vi "add-subhiearchy.vi"(6 "appended path":path, 8 "all relative paths":path[](array[path]), 9 "indices of kept elements":i32[](array[numeric]), 10 "tree main structure":string[](array[string]), 11 "all vi paths":path[](array[path])) -> ()   [LabVIEW 2014]
uses:
  controls/state-machine.ctl
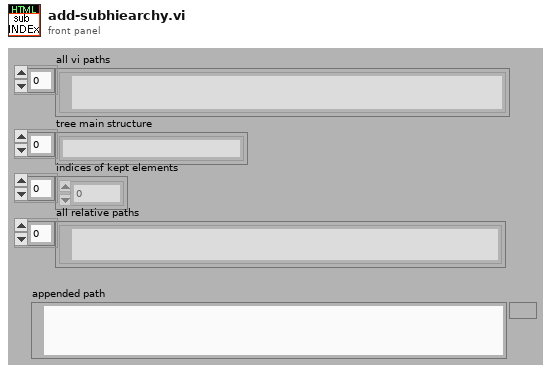
[diagram p1: front panel]
types:
  T1 = typedef "state-machine.ctl" = enum16{"add carridge return", "init", "Read-inputs", "edit generated file", "end", "Add front panel", "Add Block Diagram", "Add VI icon", "Add VI description", "Add VI hiearchy", "Add list of sub vis", "add custom html", "open report in browser", "Save report to file", "dispose report", "Add header text", "Create style .css", "add-red-box-header", "Delete Temp Files", "Remove-path-element", "add-revision-history", "add-icon-image-only"}
  T2 = typedef "state program.ctl" = cluster{"State machine":T1, "HTML before":string, "HTML after":string}
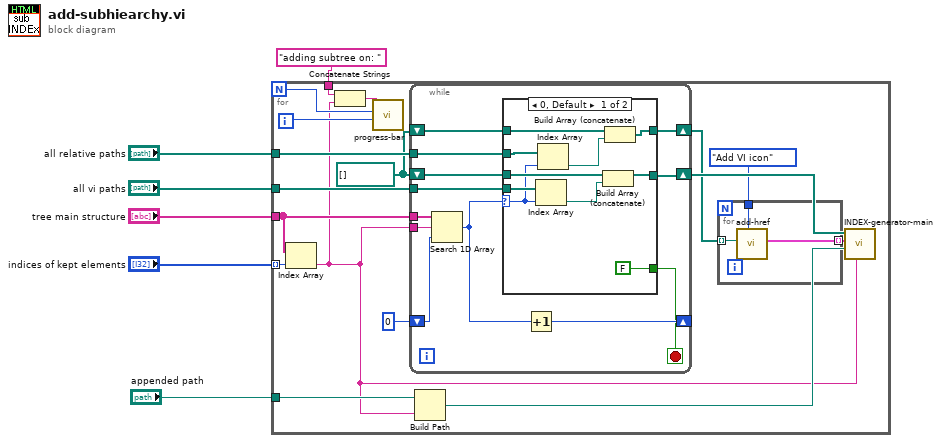
[diagram p0: block diagram]
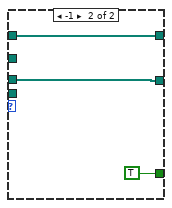
[diagram p2: hidden frame]
diagram:
  n1 = for {
    N -> [w12]
    tunnel: "tree main structure" -> [w22]
    tunnel: "indices of kept elements" -> [w23] mode=indexing
    tunnel: "all vi paths" -> [w21]
    tunnel: "all relative paths" -> [w19]
    tunnel: "appended path" -> [w15]
    tunnel: "adding subtree on: " -> [w8]
    i -> [w11]
    w18 = path[] []
    n2 = Index Array(array=w22, index=w23) -> (element=w9:string)
    n3 = Concatenate Strings(w8, w9) -> (w10:string)
    n4 = call "progress-bar.vi"("i++"=w11, "max"=w12, "state"=w10) -> ()  [unwired: 9 out]
    n5 = while {
      tunnel: w9 -> [w38]
      tunnel: w22 -> [w37]
      shift-right: [w30] -> w16
      shift-left: w18 -> [w31]
      shift-right: [w35] -> _
      shift-left: 0 -> [w36]
      tunnel: w21 -> [w32]
      shift-right: [w27] -> w13
      shift-left: w18 -> [w28]
      tunnel: w19 -> [w29]
      stop <- w33 stop-if-true
      n6 = Search 1D Array(1D array=w37, element=w38, start index (0)=w36) -> (index of element=w34:i32)
      n7 = case shown="0, Default" w34 {
        selector: w34 -> [w41 _]
        tunnel: [FALSE TRUE] -> w33
        tunnel: w32 -> [w47 _]
        tunnel: w31 -> [w45 w50]
        tunnel: [w44 w50] -> w30
        tunnel: w29 -> [w42 _]
        tunnel: w28 -> [w40 w49]
        tunnel: [w39 w49] -> w27
        frame 0, Default {
          n8 = Index Array(array=w47, index=w41) -> (element=w46:path)
          n9 = Index Array(array=w42, index=w41) -> (element=w43:path)
          n10 = Build Array (concatenate)(w45, w46) -> (w44:path[])
          n11 = Build Array (concatenate)(w40, w43) -> (w39:path[])
        }
        frame -1 {
        }
      }
      n12 = Increment(x=w34) -> (x+1=w35:i32)
    }
    n13 = Build Path(base path=w15, name or relative path=w9) -> (appended path=w14:path)
    n14 = for {
      tunnel: [w26] -> w17 mode=indexing
      tunnel: w13 -> [w25] mode=indexing
      tunnel: state-machine."Add VI icon" ("State machine") -> [w24]
      n15 = call "add-href.vi"("State machine"=w24, "relative path"=w25) -> ("state"=w26:T2)  [unwired: 9 out]
    }
    n16 = call "INDEX-generator-main.vi"("header"=w9, "report file destination"=w14, "tasks"=w17, "VI paths"=w16) -> ()  [unwired: 2 in, 6 out]
  }
